vi "2-0-Read-SRC-varid_prop.vi"(5 "prop_src (entrée)":string[](array[string]), 6 "valeurs prop (variant)":variant[](array[variant]), 7 "liste_prop":string[](array[string])) -> (2 "valeurs prop_src":string[](array[string]), 3 "prop_src (sortie)":string[](array[string]))   [LabVIEW 2010, in "lv_04.lvlib"]
uses:
  lv_04.lvlib
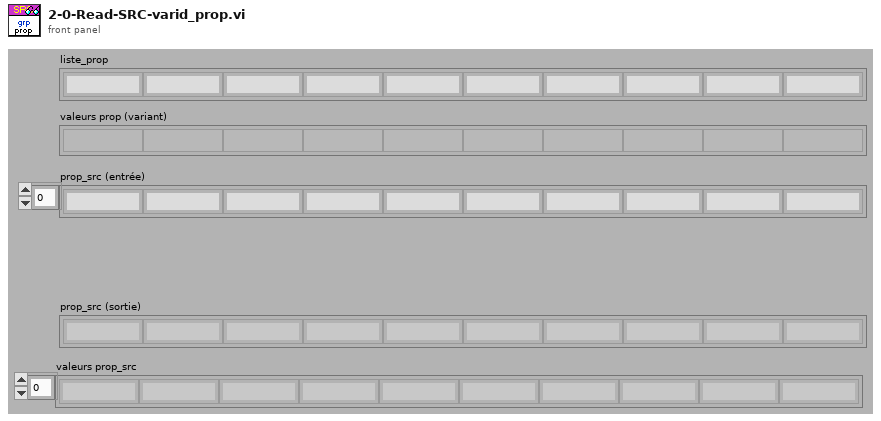
[diagram p1: front panel]
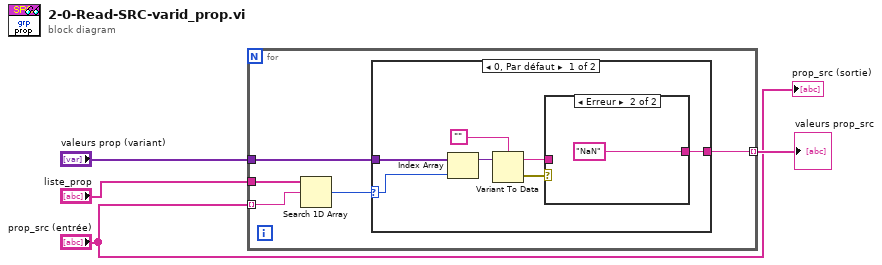
[diagram p0: block diagram]
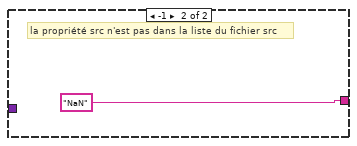
[diagram p3: hidden frame]
diagram:
  n1 = for {
    tunnel: "valeurs prop (variant)" -> [w6]
    tunnel: "liste_prop" -> [w9]
    tunnel: "prop_src (entrée)" -> [w8] mode=indexing
    tunnel: [w5] -> w2 mode=indexing
    n2 = Search 1D Array(1D array=w9, element=w8) -> (index of element=w7:i32)  [unwired: 1 in]
    n3 = case shown="0, Par défaut" w7 {
      selector: w7 -> [w12 _]
      tunnel: w6 -> [w13 _]
      tunnel: [w10 "NaN"] -> w5
      frame 0, Default {
        n4 = Index Array(array=w13, index=w12) -> (element=w11:variant)
        n5 = Variant To Data(Variant=w11, type="") -> (error out=w15:errorcluster, data=w14:string)  [unwired: 1 in]
        n6 = case shown="Erreur" w15 {
          tunnel: w14 -> [w17 _]
          tunnel: [w17 "NaN"] -> w10
          frame No Error {
          }
          frame Error {
          }
        }
      }
      frame -1 {
        # "la propriété src n'est pas dans la liste du fichier src"
      }
    }
  }
  "valeurs prop_src" <- w2
  "prop_src (sortie)" <- "prop_src (entrée)"
